vi "Teardown Created Events.vi"(11 "Base Queue in":refnum<class "Base Queue.lvclass">) -> (3 "Base Queue out":refnum<class "Base Queue.lvclass">)   [LabVIEW 2021, in "jettl.lvlib" / "Base Queue.lvlib" / "Base Queue.lvclass"]
uses:
  Base Queue.lvclass
  Base Queue.lvclass/Base Queue.ctl
  jettl Msg Teardown/jettl Msg Teardown.lvlib
  jettl Msg Teardown/Teardown Msg Strategy/Teardown Msg Strategy.lvclass
  C:/git/jettl/src/jettl Msg Teardown/Teardown Msg Strategy/Teardown Msg Strategy.lvclass
  C:/git/jettl/src/jettl/Msg Strategy/Msg Strategy.lvclass
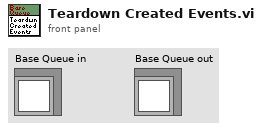
[diagram p1: front panel]
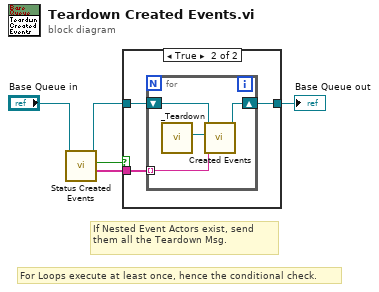
[diagram p0: block diagram]
diagram:
  # "If Nested Event Actors exist, send them all the Teardown Msg."
  # "For Loops execute at least once, hence the conditional check."
  n1 = call-dynamic "Status Created Events.vi"("Base Queue in"="Base Queue in") -> ("Created Event Aliases"=w2:string[], "Created Event Exist?"=w3:bool, "Base Queue out"=w1:refnum<class "Base Queue.lvclass">)  [unwired: 7 in, 1 out]
  n2 = case shown="True" w3 {
    tunnel: [w6 w9] -> w5
    tunnel: w1 -> [w6 w8]
    tunnel: w2 -> [_ w7]
    frame False {
    }
    frame True {
      n3 = for {
        tunnel: w7 -> [w11] mode=indexing
        shift-right: [w13] -> w9
        shift-left: w8 -> [w12]
        n4 = call "_Teardown.vi"() -> ("Teardown Msg Strategy out"=w10:refnum<class "Teardown Msg Strategy.lvclass">)  [unwired: 11 in]
        n5 = call-dynamic "Created Events.vi"("Created Event Alias"=w11, "Msg Strategy"=w10, "Base Queue in"=w12) -> ("Base Queue out"=w13:refnum<class "Base Queue.lvclass">)  [unwired: 8 in]
      }
    }
  }
  "Base Queue out" <- w5
